vi "set_outputs.vi"(11 "All_Outputs":T1) -> ()   [LabVIEW 2012]
uses:
  All_Outputs.ctl
  Cirular Shooter/Shooter_Outputs.ctl
  Climber/Climber_Outputs.ctl
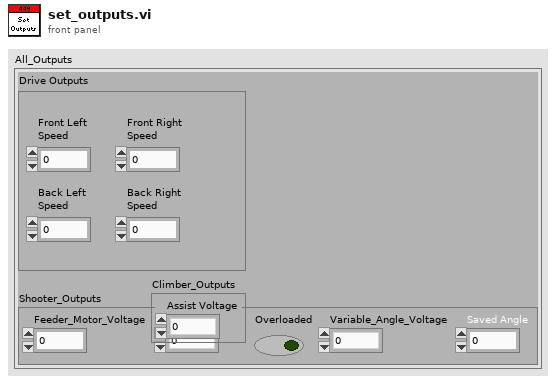
[diagram p1: front panel]
types:
  T1 = typedef "All_Outputs.ctl" = cluster{"Drive Outputs":cluster{"Front Left\nSpeed":dbl, "Back Left\nSpeed":dbl, "Front Right\nSpeed":dbl, "Back Right\nSpeed":dbl}, "Shooter_Outputs":T2, "Climber_Outputs":T3}
  T2 = typedef "Shooter_Outputs.ctl" = cluster{"Feeder_Motor_Voltage":dbl, "Output Voltage":dbl, "Overloaded":bool, "Variable_Angle_Voltage":dbl, "Saved Angle":dbl}
  T3 = typedef "Climber_Outputs.ctl" = cluster{"Assist Voltage":dbl}
  T4 = cluster{"Front Left\nSpeed":dbl, "Back Left\nSpeed":dbl, "Front Right\nSpeed":dbl, "Back Right\nSpeed":dbl}
  T5 = typedef "WPI_MotorControlDeviceRef.ctl" = cluster{"DeviceStatus":errorcluster, "Type":enum16{"PWM", "CAN"}, "PWM":cluster{"Digital Module":T6, "PWM Channel":T7, "DeadBand":T8}, "CAN":cluster{"Device Number":u8, "Control Mode":T9, "Semaphore":T10, "Max Vout":dbl}, "Invert":bool, "TransformRef":T11, "InvTransformRef":T11}
  T6 = typedef "FPGA_TypedefDigitalModule.ctl" = enum16{"Digital Module 1", "Digital Module 2"}
  T7 = typedef "FPGA_DIOPWMChannel.ctl" = enum8{"PWM 1", "PWM 2", "PWM 3", "PWM 4", "PWM 5", "PWM 6", "PWM 7", "PWM 8", "PWM 9", "PWM 10", "Invalid"}
  T8 = typedef "WPI_PWMDeadband.ctl" = cluster{"Name":string, "maxPositivePwm":i32, "minPositivePwm":i32, "centerPwm":i32, "maxNegativePwm":i32, "minNegativePwm":i32, "angularRange":u16}
  T9 = typedef "WPI_CANJaguar_ControlMode.ctl" = enum8{"Percent VBus", "Current", "Speed", "Position", "Voltage"}
  T10 = typedef "Semaphore RefNum" = refnum<k1>
  T11 = typedef "WPI_PWMTransform_ConPane.ctl" = refnum<vi>
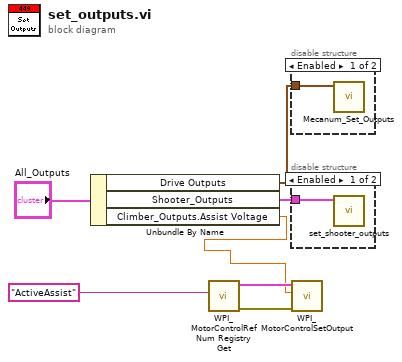
[diagram p0: block diagram]
diagram:
  n1 = Unbundle By Name("All_Outputs") -> ("Drive Outputs"=w7:T4, "Shooter_Outputs"=w5:T2, "Climber_Outputs.Assist Voltage"=w1:dbl)
  n2 = call <vilib>:"WPI_MotorControlRefNum Registry Get.vi"("refnum name"="ActiveAssist") -> ("error out"=w2:errorcluster, "MotorControlDevRef"=w3:T5)  [unwired: 9 in]
  n3 = disable-structure shown="Enabled" {
    disable-tunnel: w7 -> [w8 _]
    frame Enabled {
      n4 = call "Mecanum_Set_Outputs.vi"("Drive Outputs"=w8) -> ()  [unwired: 11 in]
    }
    frame Disabled {
    }
  }
  n5 = disable-structure shown="Enabled" {
    disable-tunnel: w5 -> [w9 _]
    frame Enabled {
      n6 = call "set_shooter_outputs.vi"("Shooter_Outputs"=w9) -> ()  [unwired: 11 in]
    }
    frame Disabled {
    }
  }
  n7 = call <vilib>:"WPI_MotorControlSetOutput.vi"("error in (no error)"=w2, "Output"=w1, "MotorControlDevRef"=w3) -> ()  [unwired: 6 in, 3 out]
